vi "main.vi"() -> ()   [LabVIEW 2016]
uses:
  stages.ctl
panel:
  in  "Sawtooth Wave Duration":dbl=20.0 format="%.2f"
  in  "Sawtooth Wave Oscillations":dbl=10.0 format="%.2f"
  out "Frequency":dbl=0.5 format="%.2f"
  in  "Sawtooth Wave Amplitude":dbl=3.0 format="%0.2f"
  in  "Sawtooth Wave DC Offset":dbl=4.0 format="%0.2f"
  in  "Hold1 Duration":dbl=2.0
  in  "Hold1 DC Offset":dbl
  in  "Sine Wave DC Offset":dbl=7.0 format="%0.2f"
  in  "Sine Wave Amplitude":dbl=1.0 format="%0.2f"
  in  "Square Wave DC Offset":dbl=4.0 format="%0.2f"
  in  "Square Wave Amplitude":dbl=3.0 format="%0.2f"
  in  "stop":bool
  in  "Hold DC Offset":dbl=3.0
  in  "Hold Duration":dbl=8.0
  in  "Ramp Amplitude":dbl=10.0
  in  "Ramp Duration":dbl=8.0
  out "Frequency":dbl=0.5 format="%.2f"
  in  "Square Wave Duration (s)":dbl=20.0 format="%.2f"
  in  "Square Wave Oscillations":dbl=10.0 format="%.2f"
  in  "Sine Wave Duration":dbl=14.0 format="%.2f"
  in  "Sine Wave Oscillations":dbl=10.0 format="%.2f"
  out "Frequency":dbl=0.5 format="%.2f"
  out "Output Waveform":cluster{"frequency":dbl, dbl, dbl[]}(graph)={"frequency"=0.0, 0.001, []}
  in  "Sampling Rate (Hz)":dbl(slide)=1000.0 scale=0.0..1000.0
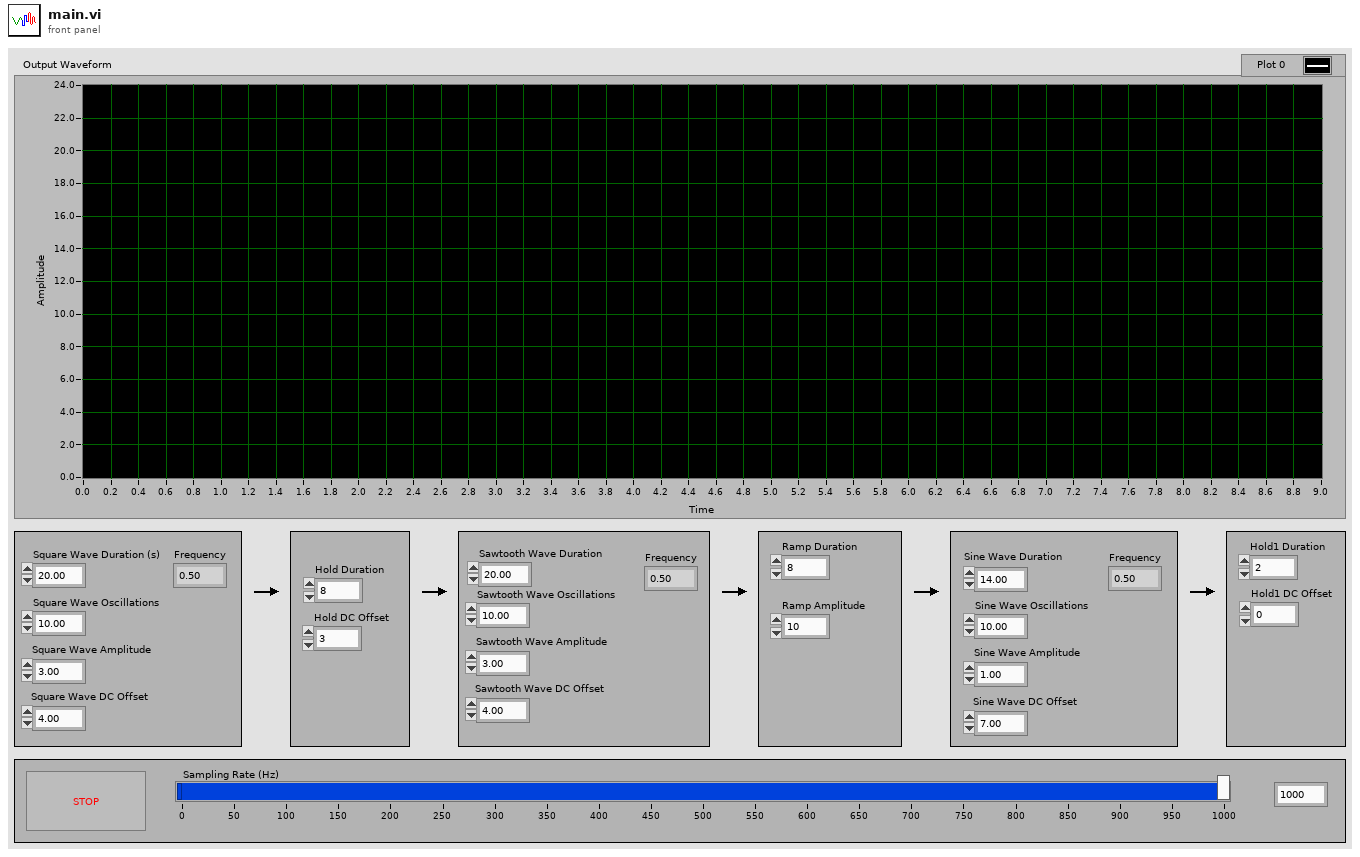
[diagram p1: front panel]
types:
  T1 = typedef "stages.ctl" = enum16{"Stop", "Hold1", "SawtoothWave", "SineWave", "Hold2", "Hold", "Ramp", "SquareWave", "Initialisation"}
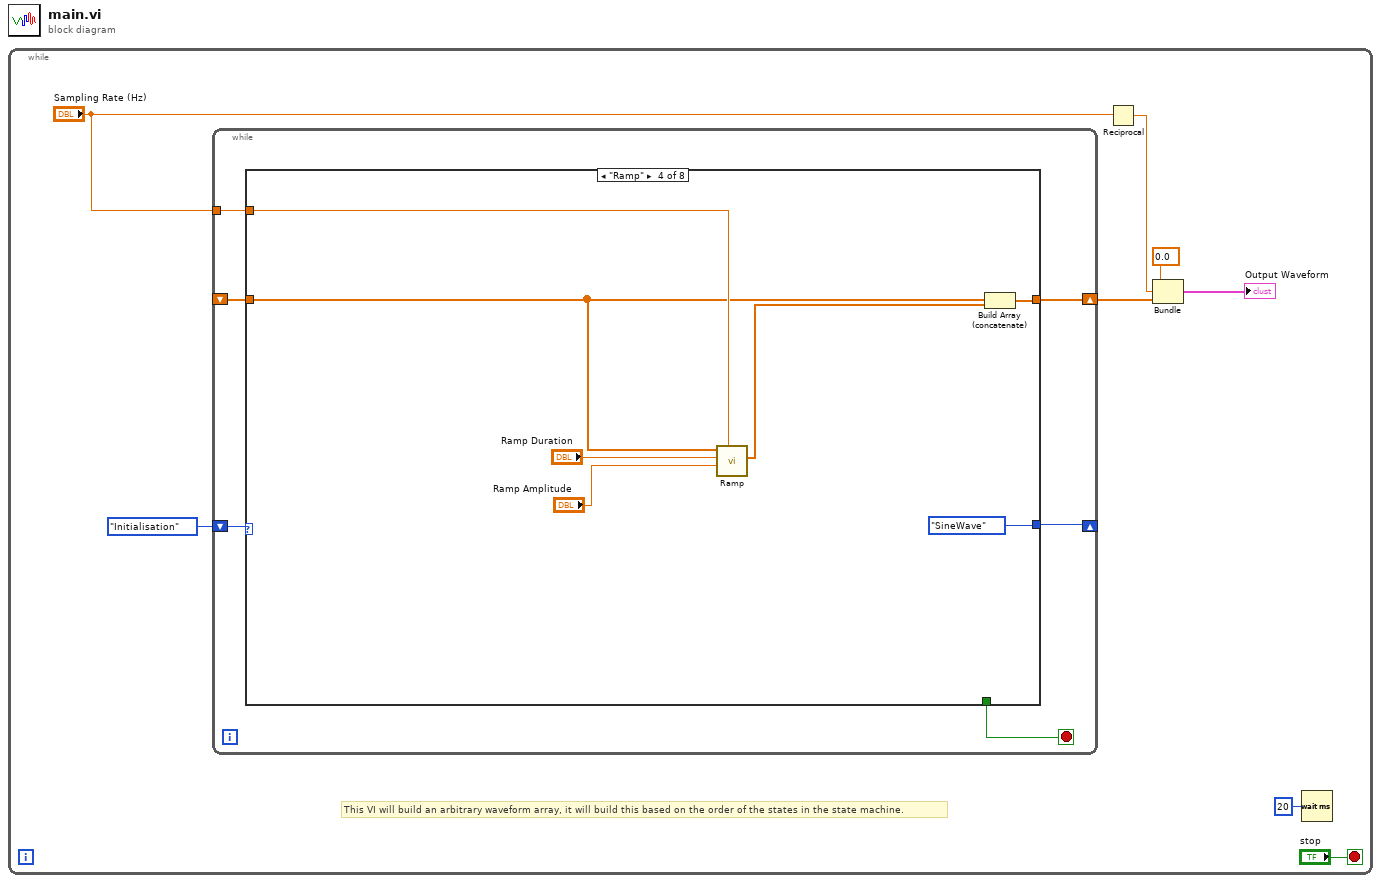
[diagram p0: block diagram]
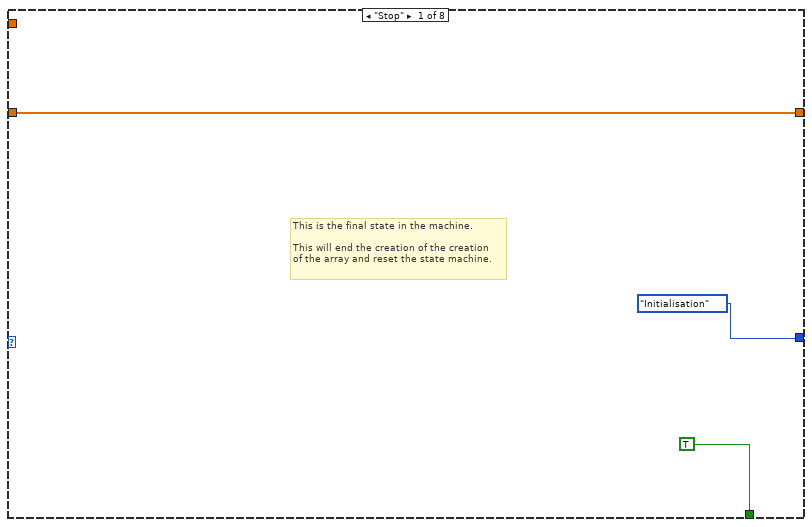
[diagram p2: hidden frame]
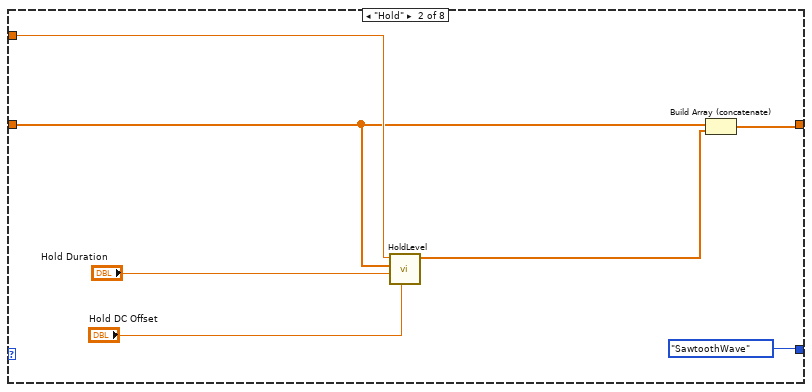
[diagram p3: hidden frame]
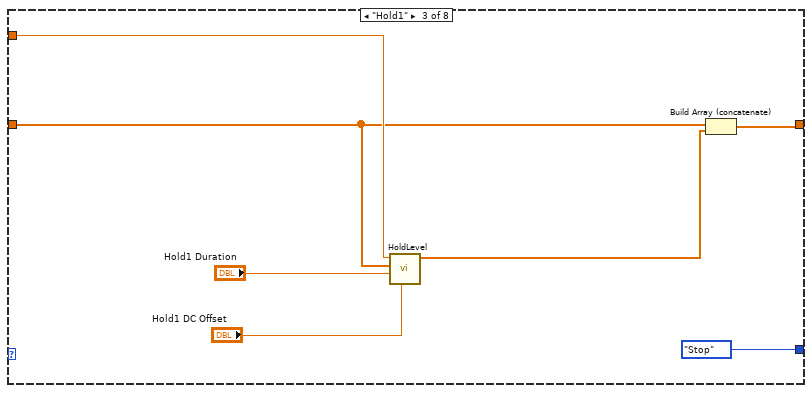
[diagram p4: hidden frame]
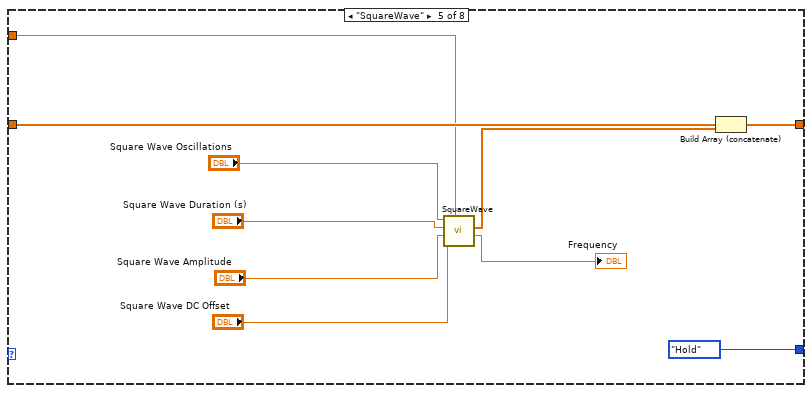
[diagram p5: hidden frame]
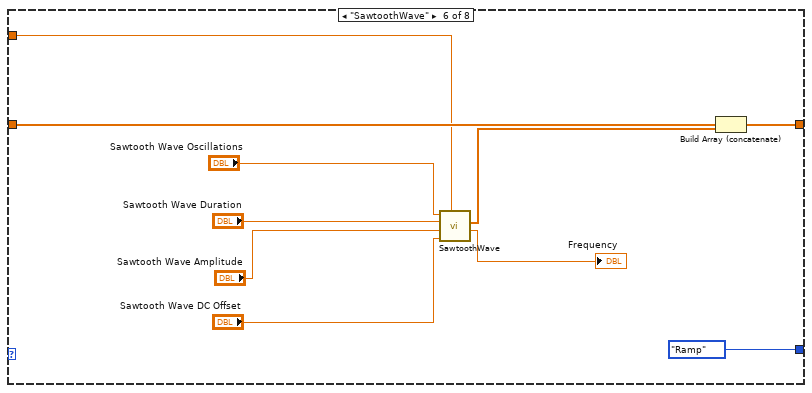
[diagram p6: hidden frame]
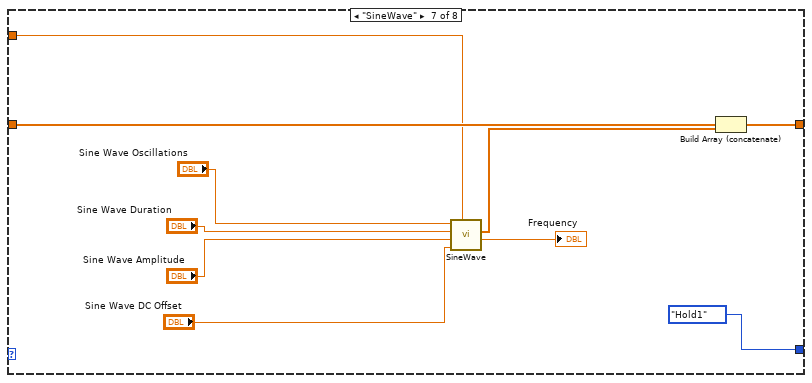
[diagram p7: hidden frame]
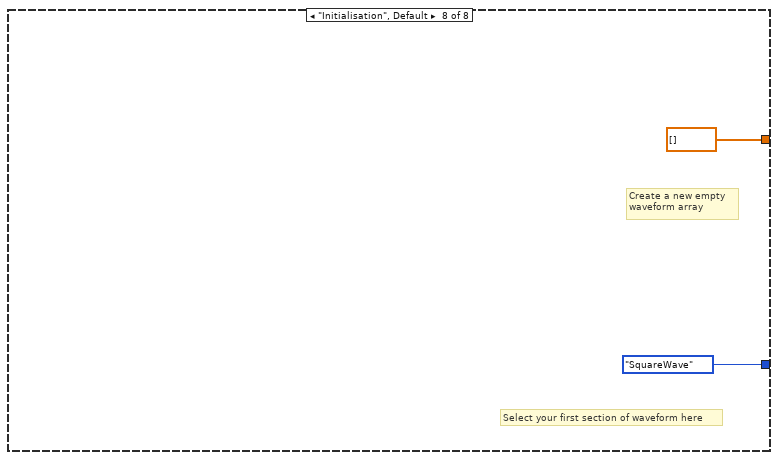
[diagram p8: hidden frame]
diagram:
  n1 = while {
    stop <- "stop" stop-if-true
    # "This VI will build an arbitrary waveform array, it will build this based on the order of the states in the state machine."
    n2 = while {
      shift-right: [w13] -> _
      shift-left: stages."Initialisation" -> [w14]
      shift-right: [w11] -> w6
      shift-left: _ -> [w10]
      tunnel: "Sampling Rate (Hz)" -> [w9]
      stop <- w12 stop-if-true
      n3 = case shown="\"Ramp\"" w14 {
        tunnel: [stages."Initialisation" stages."SawtoothWave" stages."Stop" stages."SineWave" stages."Hold" stages."Ramp" stages."Hold1" stages."SquareWave"] -> w13
        tunnel: [TRUE _ _ _ _ _ _ _] -> w12
        tunnel: [w15 w23 w30 w37 w46 w56 w66 dbl[] []] -> w11
        tunnel: w10 -> [w15 w20 w27 w34 w47 w57 w67 _]
        tunnel: w9 -> [_ w21 w28 w36 w43 w55 w65 _]
        frame "Stop" {
          # "This is the final state in the machine.\n\nThis will end the creation of the creation\nof the array and reset the state machine."
        }
        frame "Hold" {
          n4 = call "HoldLevel.vi"("Hold DC Offset"="Hold DC Offset", "Hold Duration"="Hold Duration", "SignalIn"=w20, "Sample Rate"=w21) -> ("SignalOut"=w19:dbl[])  [unwired: 7 in]
          n5 = Build Array (concatenate)(w20, w19) -> (w23:dbl[])
        }
        frame "Hold1" {
          n6 = call "HoldLevel.vi"("Hold DC Offset"="Hold1 DC Offset", "Hold Duration"="Hold1 Duration", "SignalIn"=w27, "Sample Rate"=w28) -> ("SignalOut"=w26:dbl[])  [unwired: 7 in]
          n7 = Build Array (concatenate)(w27, w26) -> (w30:dbl[])
        }
        frame "Ramp" {
          n8 = call "Ramp.vi"("Sample Rate"=w36, "Ramp Amplitude"="Ramp Amplitude", "Ramp Duration"="Ramp Duration", "Array in"=w34) -> ("Array out"=w35:dbl[])  [unwired: 7 in]
          n9 = Build Array (concatenate)(w34, w35) -> (w37:dbl[])
        }
        frame "SquareWave" {
          n10 = call "SquareWave.vi"("Sample Rate"=w43, "Sawtooth Wave DC Offset"="Square Wave DC Offset", "Sawtooth Wave Amplitude"="Square Wave Amplitude", "Sawtooth Wave Duration"="Square Wave Duration (s)", "Sawtooth Wave Oscillations"="Square Wave Oscillations") -> ("Frequency"=→"Frequency":dbl, "signal"=w45:dbl[])  [unwired: 5 in]
          n11 = Build Array (concatenate)(w47, w45) -> (w46:dbl[])
        }
        frame "SawtoothWave" {
          n12 = call "SawtoothWave.vi"("Sample Rate"=w55, "Sawtooth Wave DC Offset"="Sawtooth Wave DC Offset", "Sawtooth Wave Amplitude"="Sawtooth Wave Amplitude", "Sawtooth Wave Duration"="Sawtooth Wave Duration", "Sawtooth Wave Oscillations"="Sawtooth Wave Oscillations") -> ("Frequency"=→"Frequency":dbl, "signal"=w50:dbl[])  [unwired: 5 in]
          n13 = Build Array (concatenate)(w57, w50) -> (w56:dbl[])
        }
        frame "SineWave" {
          n14 = call "SineWave.vi"("Sample Rate"=w65, "Sine Wave DC Offset"="Sine Wave DC Offset", "Sine Wave Amplitude"="Sine Wave Amplitude", "Sine Wave Duration"="Sine Wave Duration", "Sine Wave Oscillations"="Sine Wave Oscillations") -> ("Frequency"=→"Frequency":dbl, "signal"=w59:dbl[])  [unwired: 5 in]
          n15 = Build Array (concatenate)(w67, w59) -> (w66:dbl[])
        }
        frame "Initialisation", Default {
          # "Create a new empty \nwaveform array"
          # "Select your first section of waveform here"
        }
      }
    }
    n16 = Reciprocal(x="Sampling Rate (Hz)") -> (1/x=w3:dbl)
    n17 = Bundle("frequency"=0.0, w3, w6) -> (→"Output Waveform":cluster{"frequency":dbl, dbl, dbl[]})  [unwired: 1 in]
    n18 = Wait (ms)(milliseconds to wait=u32 20) -> ()  [unwired: 1 out]
  }
